vi "flushStackTubing.vi"(8 "measQ":dbl, 10 "Traverse line":T2 {"Carrier_2 Q (l/min)" format="%#.2f"; "Row Duration (mins)" format="%#.1f"; "Row No" min=0; "Trace Gas Concentration (%)" min=0.0 format="%#_4f"; "Carrier_1 Q (l/min)" format="%#.4f"; "Start X" format="%#.2f"; "Start Y" format="%#.2f"; "Start Z" format="%#.2f"; "End X" format="%#.2f"; "End Y" format="%#.2f"; "End Z" format="%#.2f"; "Tunnel Speed" format="%#.2f"; "Averaging time (mins)" min=0.0 format="%#.2f"}, 11 "Simulate/Run":T1) -> (1 "endTime":dbl)   [LabVIEW 2021]
uses:
  Gen Trav/Traverse_cluster.ctl
  Gen Trav/Spacing.ctl
  Controls/Multi_run_mode.ctl
  Controls/User_Specific_mode.ctl
  03d3161e-5303-a34a-bfc6-4d490536d823.vi
panel:
  out "flushTime(s)":dbl
  in  "nPurges":dbl=10.0 format="%#_13g"
  in  "stackTubeVolume(l)":dbl=3.0 format="%#_13g"
  # "X           Y          Z"
  # "Start"
  # "End"
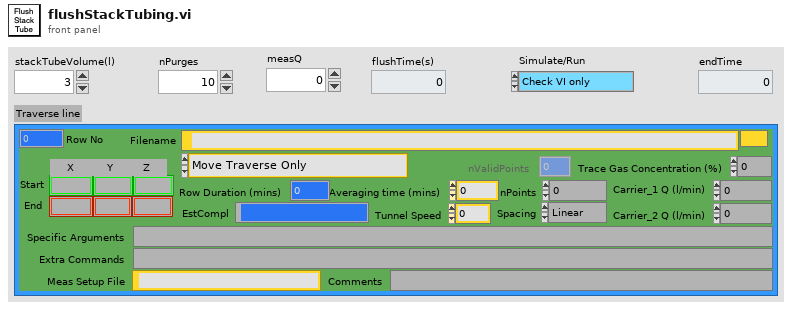
[diagram p1: front panel]
types:
  T1 = typedef "User_Specific_mode.ctl" = enum16{"Check VI only", "Run VI"}
  T2 = typedef "Traverse_cluster.ctl" = cluster{"Start X":sgl, "Start Y":sgl, "Start Z":sgl, "End X":sgl, "End Y":sgl, "End Z":sgl, "nPoints":i32, "Spacing":T3, "Filename":path, "Tunnel Speed":dbl, "Averaging time (mins)":dbl, "Extra Commands":string, "Carrier_1 Q (l/min)":dbl, "Carrier_2 Q (l/min)":dbl, "Trace Gas Concentration (%)":dbl, "Specific Arguments":string, "Comments":string, "Row No":i32, "Row Type Selector":T4, "EstCompl":string, "Row Duration (mins)":dbl, "nValidPoints":i32, "Meas Setup File":string}
  T3 = typedef "Spacing.ctl" = enum16{"Linear", "Log", "Gauss", "Specified", "N/A"}
  T4 = typedef "Multi_run_mode.ctl" = enum16{"Move Traverse Only", "Set Tunnel Speed Only", "Set Source Only", "Set Measurement Conditions", "Single Measurement", "Vertical Profile", "Lateral Profile", "Longitudinal Profile", "Multi-Axis Profile", "Explore Volume", "Auto Calibrate", "Meas Fast FID Bkgnd", "Check Beam Power", "Scanning Valve Measurement", "Run VI Named:", "Set ADAM Ch", "Wait (minutes)", "Send Message", "Synchronize With:", "Fall Back to this Row", "Turn Off Row Repeating", "Traverse 3D Volume", "Blank Row", "Jump to Fall Back Row"}
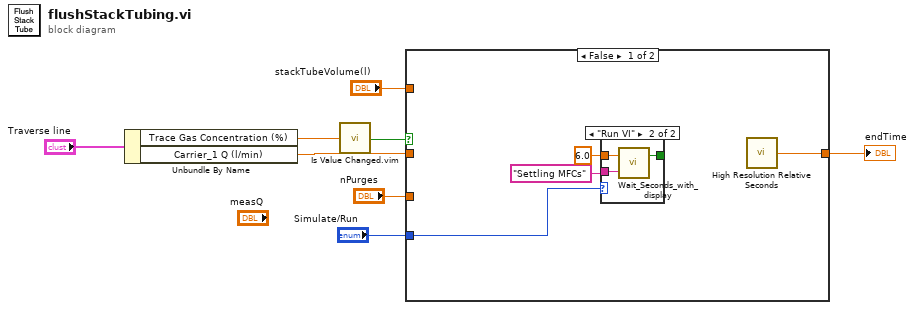
[diagram p0: block diagram]
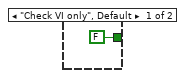
[diagram p2: hidden frame]
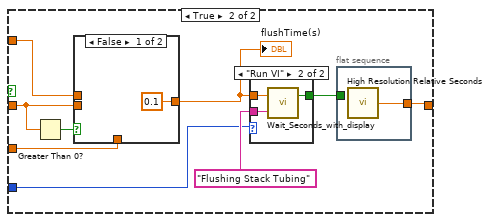
[diagram p3: hidden frame]
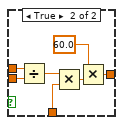
[diagram p4: hidden frame]
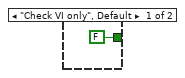
[diagram p5: hidden frame]
diagram:
  n1 = Unbundle By Name("Traverse line") -> ("Trace Gas Concentration (%)"=w7:dbl, "Carrier_1 Q (l/min)"=w8:dbl)
  n2 = call "Is Value Changed.vim"("value"=w7) -> ("changed or first call?"=w5:bool)
  n3 = case shown="False" w5 {
    tunnel: [w12 w23] -> w4
    tunnel: w8 -> [_ w17]
    tunnel: "stackTubeVolume(l)" -> [_ w21]
    tunnel: "nPurges" -> [_ w20]
    tunnel: "Simulate/Run" -> [w11 w19]
    frame False {
      n4 = case shown="\"Run VI\"" w11 {
        tunnel: "Settling MFCs" ("Message") -> [_ w16]
        tunnel: [FALSE ("Stopped") w15] -> _
        tunnel: 6.0 -> [_ w14]
        frame "Check VI only", Default {
        }
        frame "Run VI" {
          n5 = call "Wait_Seconds_with_display.vi"("Message"=w16, "Seconds to wait"=w14) -> ("Stopped"=w15:bool)  [unwired: 1 out]
        }
      }
      n6 = call <vilib>:"High Resolution Relative Seconds.vi"() -> ("relative seconds"=w12:dbl)
    }
    frame True {
      n7 = Greater Than 0?(x=w17) -> (x > 0?=w18:bool)
      n8 = case shown="False" w18 {
        tunnel: [0.1 w31] -> w22
        tunnel: w17 -> [_ w29]
        tunnel: w21 -> [_ w28]
        tunnel: w20 -> [_ w27]
        frame False {
        }
        frame True {
          n9 = Divide(x=w28, y=w29) -> (x/y=w33:dbl)
          n10 = Multiply(x=w33, y=w27) -> (x*y=w32:dbl)
          n11 = Multiply(x=60.0, y=w32) -> (x*y=w31:dbl)
        }
      }
      "flushTime(s)" <- w22
      n12 = case shown="\"Run VI\"" w19 {
        tunnel: "Flushing Stack Tubing" ("Message") -> [_ w37]
        tunnel: [FALSE ("Stopped") w36] -> w24
        tunnel: w22 -> [_ w35]
        frame "Check VI only", Default {
        }
        frame "Run VI" {
          n13 = call "Wait_Seconds_with_display.vi"("Message"=w37, "Seconds to wait"=w35) -> ("Stopped"=w36:bool)  [unwired: 1 out]
        }
      }
      n14 = flat-sequence {
        tunnel: w24 -> [_]
        tunnel: [w38] -> w23
        frame #0 {
          n15 = call <vilib>:"High Resolution Relative Seconds.vi"() -> ("relative seconds"=w38:dbl)
        }
      }
    }
  }
  "endTime" <- w4
